vi "Update Plot.vi"(0 "Display State In":T1, 5 "plotnum":i32, 7 "plot":cluster{"X":dbl[], "Y":dbl[]}, 9 "Container State":T6, 11 "error in (no error)":errorcluster, 12 "color":u32(colorbox)=16777216, 13 "name":string) -> (4 "Display State Out":T1, 15 "error out":errorcluster)   [LabVIEW 2015, in "Interactive Graph.xctl"]
uses:
  Interactive Graph.xctl
  <vilib>/_xctls/Container State.ctl
  State.vi
  Persistent.ctl
  Plot.ctl
  EPhys/LV Source/Work Panel VIs/Typedefs/EPhysWork-Label Position.ctl
  Events.ctl
  Selection.ctl
  XRange.ctl
  YScale.ctl
  Cursor.ctl
  <vilib>/_xctls/XControlSupport.lvlib
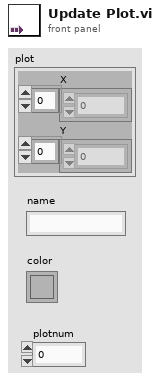
[diagram p1: front panel]
types:
  T1 = typedef "Interactive Graph.xctl/State.vi" = cluster{"ref":refnum<vi>, "actions":string[], "Persist":T2, "cursor":bool, "prescale":dbl, "palette":u32[], "colIndex":i32, "to add":T3, "Events":T5, "selected":i32, "to show":cluster{"Visible":bool, "Start":i32, "Length":i32}, "maxplot":i32, "Y0":dbl[], "plotnum":i32}
  T2 = typedef "Interactive Graph.xctl/Persistent.ctl" = cluster{"Scale":dbl, "Xrange":cluster{"min":dbl, "max":dbl}}
  T3 = typedef "Interactive Graph.xctl/Plot.ctl" = cluster{"plot":cluster{"X":dbl[], "Y":dbl[]}, "name":string, "Y0":dbl, "color":u32, "Style":enum16{"Normal", "Highlight", "Shadow"}, "labpos":T4, "visible":bool, "cursor":bool}
  T4 = typedef "EPhysWork-Label Position.ctl" = cluster{"Index":i32, "Xoff":dbl, "Yoff":dbl}
  T5 = typedef "Interactive Graph.xctl/Events.ctl" = cluster{"Selection":refnum<user-event>, "XRange":refnum<user-event>, "YScale":refnum<user-event>, "CursorPos":refnum<user-event>}
  T6 = typedef "XControlSupport.lvlib/Container State.ctl" = cluster{"Indicator?":bool, "Run Mode?":bool, " Refnum":refnum<vi>}
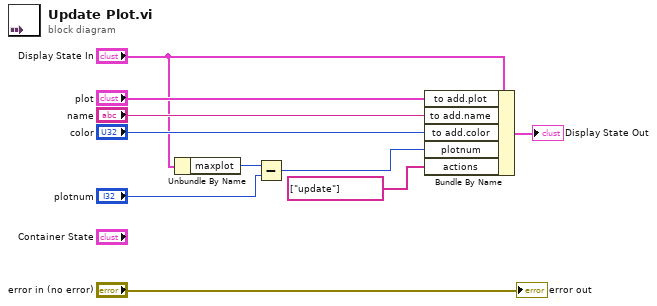
[diagram p0: block diagram]
diagram:
  n1 = Unbundle By Name("Display State In") -> ("maxplot"=w7:i32)
  n2 = Subtract(x=w7, y="plotnum") -> (x-y=w8:i32)
  n3 = Bundle By Name(cluster="Display State In", "to add.plot"="plot", "to add.name"="name", "to add.color"="color", "plotnum"=w8, "actions"=string[] ["update"]) -> (→"Display State Out":T1)
  "error out" <- "error in (no error)"
